vi "Initialize.vi"(8 "error in (no error)":errorcluster, 11 "View Template in":refnum<class "[V] Waveform.lvclass">) -> (0 "error out":errorcluster, 3 "View Template out":refnum<class "[V] Waveform.lvclass">)   [LabVIEW 2020, in "[V] Waveform.lvlib" / "[V] Waveform.lvclass"]
uses:
  [V] Waveform.lvclass
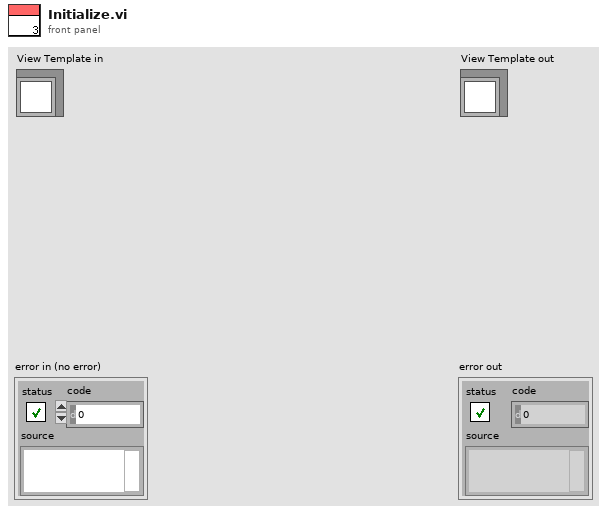
[diagram p1: front panel]
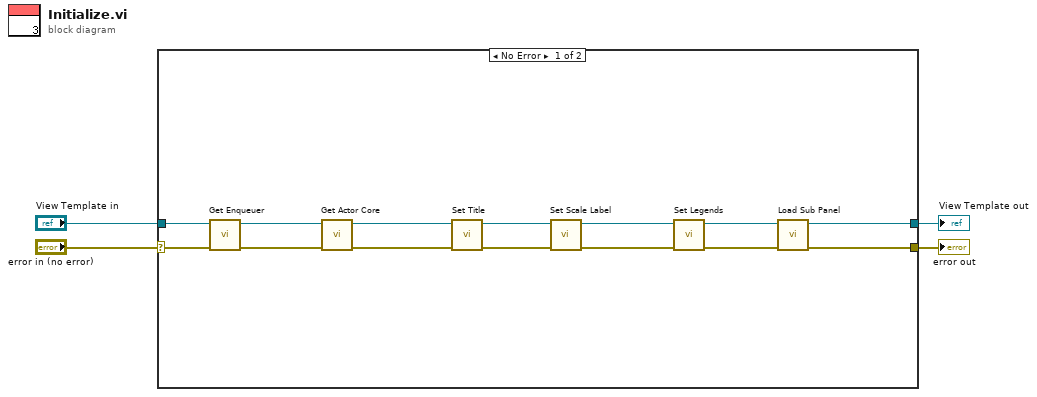
[diagram p0: block diagram]
diagram:
  n1 = case shown="No Error" "error in (no error)" {
    selector: "error in (no error)" -> [w17 w20]
    tunnel: [w5 w20] -> w3
    tunnel: [w6 w19] -> w1
    tunnel: "View Template in" -> [w18 w19]
    frame No Error {
      n2 = call "Get Enqueuer.vi"("error in (no error)"=w17, "View Template in"=w18) -> ("error out"=w16:errorcluster, "View Template out"=w15:refnum<class "[V] Waveform.lvclass">)  [unwired: 8 in]
      n3 = call "Get Actor Core.vi"("error in (no error)"=w16, "[V] Waveform in"=w15) -> ("error out"=w13:errorcluster, "[V] Waveform out"=w14:refnum<class "[V] Waveform.lvclass">)  [unwired: 8 in]
      n4 = call "Set Title.vi"("error in (no error)"=w13, "[V] Waveform in"=w14) -> ("error out"=w11:errorcluster, "[V] Waveform out"=w12:refnum<class "[V] Waveform.lvclass">)  [unwired: 8 in]
      n5 = call "Set Scale Label.vi"("error in (no error)"=w11, "[V] Waveform in"=w12) -> ("error out"=w9:errorcluster, "[V] Waveform out"=w10:refnum<class "[V] Waveform.lvclass">)  [unwired: 8 in]
      n6 = call "Set Legends.vi"("error in (no error)"=w9, "[V] Waveform in"=w10) -> ("error out"=w7:errorcluster, "[V] Waveform out"=w8:refnum<class "[V] Waveform.lvclass">)  [unwired: 8 in]
      n7 = call "Load Sub Panel.vi"("error in (no error)"=w7, "[V] Waveform in"=w8) -> ("error out"=w5:errorcluster, "[V] Waveform out"=w6:refnum<class "[V] Waveform.lvclass">)  [unwired: 8 in]
    }
    frame Error {
    }
  }
  "error out" <- w3
  "View Template out" <- w1
